vi "PicamParameters.vi"() -> ()   [LabVIEW 2019]
panel:
  in  "Cluster":T1
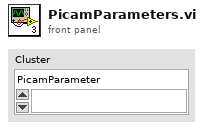
[diagram p1: front panel]
types:
  T1 = cluster{"PicamParameter":enum32{"", "SensorTemperatureReading"}}
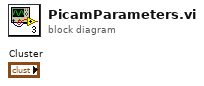
[diagram p0: block diagram]
diagram:
